vi "ACK.vi"(8 "error in (no error)":errorcluster, 11 "TCP Network Connection in":refnum<k5>) -> (0 "error out":errorcluster, 2 "Command Status":bool, 3 "TCP Network Connection out":refnum<k5>)   [LabVIEW 2019]
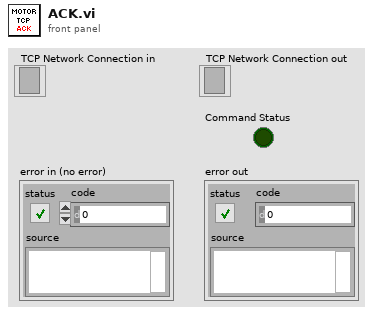
[diagram p1: front panel]
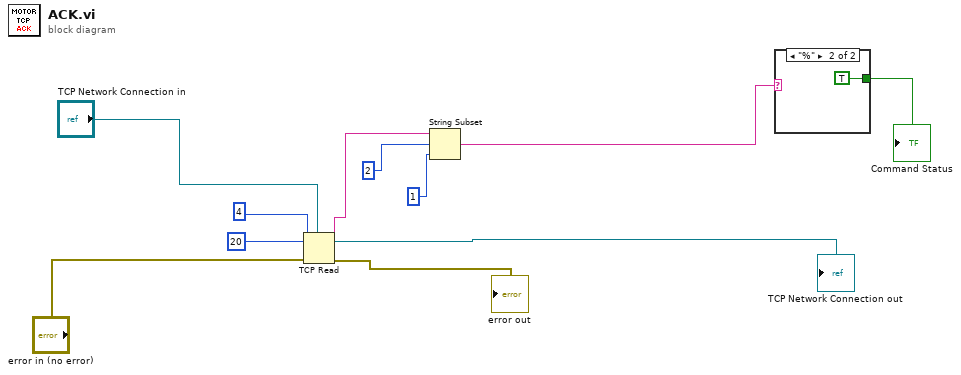
[diagram p0: block diagram]
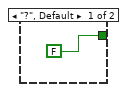
[diagram p2: hidden frame]
diagram:
  n1 = TCP Read(connection ID="TCP Network Connection in", bytes to read=4, error in (no error)="error in (no error)", 9:20 ("timeout ms (25000)")) -> (connection ID out=→"TCP Network Connection out":refnum<k5>, data out=w4:string, error out=→"error out":errorcluster)  [unwired: 1 in]
  n2 = String Subset(string=w4, offset (0)=2, length (rest)=1 ("length (rest)")) -> (substring=w5:string)
  n3 = case shown="\"%\"" w5 {
    tunnel: [FALSE ("Command Executed 2") TRUE ("Command Executed 2")] -> w10
    frame "?", Default {
    }
    frame "%" {
    }
  }
  "Command Status" <- w10
